vi "RESTFul Check_ASCII.vi"(8 "error in (no error)":errorcluster, 11 "string in":string) -> (0 "error out":errorcluster, 1 "invalid chars?":bool)   [LabVIEW 2020]
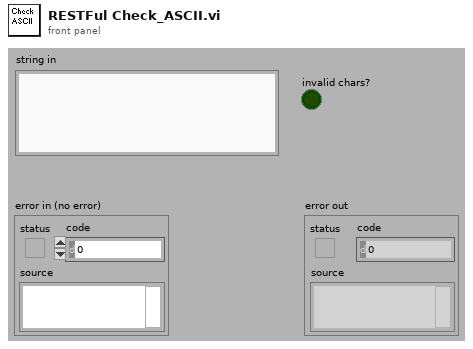
[diagram p1: front panel]
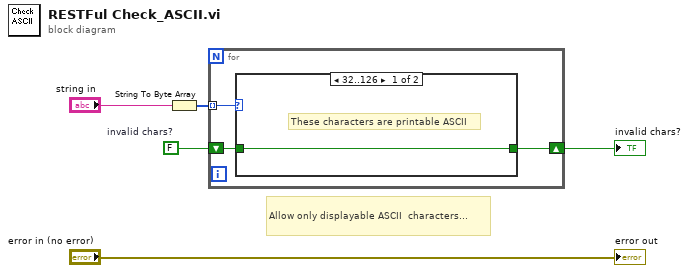
[diagram p0: block diagram]
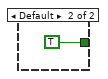
[diagram p2: hidden frame]
diagram:
  w2 = FALSE  # invalid chars?
  # "Allow only displayable ASCII  characters..."
  n1 = String To Byte Array(string="string in") -> (unsigned byte array=w3:u8[])
  n2 = for {
    tunnel: w3 -> [w8] mode=indexing
    shift-right: [w7] -> w5
    shift-left: w2 -> [w6]
    n3 = case shown="32..126" w8 {
      tunnel: [w9 TRUE ("invalid chars?")] -> w7
      tunnel: w6 -> [w9 _]
      frame 32..126 {
        # "These characters are printable ASCII"
      }
      frame Default {
      }
    }
  }
  "invalid chars?" <- w5
  "error out" <- "error in (no error)"
